vi "649SetFinal copy.vi"() -> ()   [LabVIEW 2023]
uses:
  <vilib>/numeric/Random Number (Range) U64.vi
  <vilib>/numeric/sub_Random U32.vi
  <vilib>/Utility/file.llb/Write Delimited Spreadsheet (I64).vi
  <vilib>/Utility/file.llb/Write Delimited Spreadsheet (string).vi
panel:
  out "error out":errorcluster
  in  "File path":path
  out "?":string[](array[string])
  out "?":string[][](array[string])
  in  "?":bool
  # "6@49"
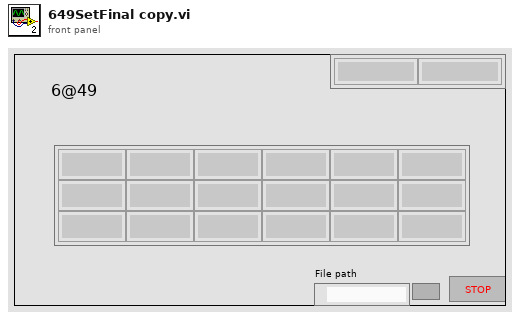
[diagram p1: front panel]
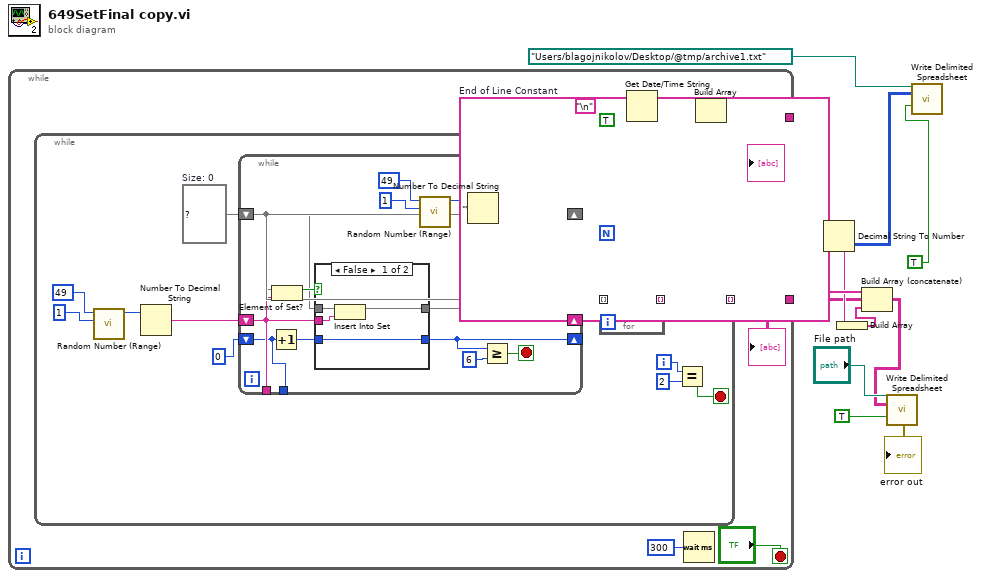
[diagram p0: block diagram]
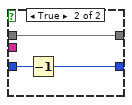
[diagram p2: hidden frame]
diagram:
  w8 = "\n"  # End of Line Constant
  n1 = while {
    tunnel: [w19] -> w2
    tunnel: [w13] -> w11
    stop <- "?" stop-if-true
    n2 = while {
      tunnel: [w20] -> w19 mode=indexing
      i -> [w25]
      stop <- w23 stop-if-true
      w30 = set{string} {}  # Size: 0
      n3 = call-poly <vilib>:"Random Number (Range).vi"("lower bound (0)"=u64 1, "upper bound (100)"=u64 49) -> ("number"=w27:u64)  [unwired: 9 in]
      n4 = Number To Decimal String(number=w27) -> (decimal integer string=w26:string)  [unwired: 1 in]
      n5 = while {
        shift-right: [w36] -> _
        shift-left: w26 -> [w33]
        shift-right: [w42] -> w21
        shift-left: w30 -> [w43]
        shift-right: [w35] -> _
        shift-left: 0 -> [w32]
        tunnel: [w33] -> _
        tunnel: [w32] -> _
        stop <- w41 stop-if-true
        n6 = Increment(x=w32) -> (x+1=w34:i32)
        n7 = Element of Set?(10:w33, 11:w43) -> (3:w44:bool)
        n8 = case shown="False" w44 {
          tunnel: w43 -> [w48 w51]
          tunnel: [w47 w51] -> w42
          tunnel: w34 -> [w46 w50]
          tunnel: [w46 w49] -> w35
          tunnel: w33 -> [w45 _]
          frame False {
            n9 = Insert Into Set(10:w45, 11:w48) -> (3:w47:set{string})  [unwired: 1 out]
          }
          frame True {
            n10 = Decrement(x=w50) -> (x-1=w49:i32)
          }
        }
        n11 = call-poly <vilib>:"Random Number (Range).vi"("lower bound (0)"=u64 1, "upper bound (100)"=u64 49) -> ("number"=w37:u64)  [unwired: 9 in]
        n12 = Number To Decimal String(number=w37) -> (decimal integer string=w36:string)  [unwired: 1 in]
        n13 = Greater Or Equal?(x=w35, y=6) -> (x >= y?=w41:bool)
      }
      n14 = for {
        tunnel: [w31] -> w20 mode=indexing
        tunnel: w21 -> [w31] mode=indexing
      }
      n15 = Equal?(x=w25, y=2) -> (x = y?=w23:bool)
    }
    "?" <- w19
    n16 = Get Date/Time String(want seconds? (F)=TRUE) -> (date string=w15:string, time string=w16:string)  [unwired: 2 in]
    n17 = Wait (ms)(milliseconds to wait=u32 300) -> ()  [unwired: 1 out]
    n18 = Build Array(w15, w16, "\n") -> (w13:string[])
    "?" <- w13
  }
  n19 = Decimal String To Number(string=w2) -> (number=w1:i32[][])  [unwired: 2 in, 1 out]
  n20 = Build Array(w8) -> (w7:string[])
  n21 = Build Array (concatenate) "Build Array"(w11, w2, w7) -> (w5:string[][])
  n22 = call-poly <vilib>:"Write Delimited Spreadsheet.vi"("file path (dialog if empty)"="File path", "2D data"=w5, "append to file? (new file:F)"=TRUE) -> ("error out"=→"error out":errorcluster)  [unwired: 11 in, 1 out]
  n23 = call-poly <vilib>:"Write Delimited Spreadsheet.vi"("file path (dialog if empty)"=path "/Users/blagojnikolov/Desktop/@tmp/archive1.txt", "2D data"=w1, "append to file? (new file:F)"=TRUE) -> ()  [unwired: 11 in, 2 out]
